vi "PPMS2 Client.vi"(8 "error in (no error)":errorcluster, 9 "Data":variant, 10 "Command":T1, 11 "instrument.PPMS2 in":refnum<class "instrument.PPMS2.lvclass">) -> (0 "error out":errorcluster, 1 "Data out":variant, 2 "Command out":string, 3 "instrument.PPMS2 out":refnum<class "instrument.PPMS2.lvclass">)   [LabVIEW 2016, in "instrument.PPMS2.lvclass"]
uses:
  instrument.PPMS2.lvclass
  C:/Program Files (x86)/National Instruments/LabVIEW 2016/user.lib/LevyLab/Levylab Instruments/SMOs/Instrument/Instrument.lvclass
  Typedefs/Commands-enum.ctl
  <userlib>/LevyLab/Levylab Instruments/SMOs/Instrument/Instrument.lvclass
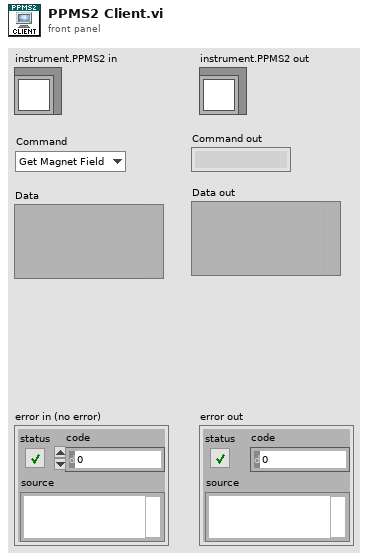
[diagram p1: front panel]
types:
  T1 = typedef "instrument.PPMS2.lvclass/Commands-enum.ctl" = enum16{"Get Magnet Field", "Get Helium Level", "Get Temperature", "Get Angle", "Set Magnet Field", "Set Temperature", "Set Angle", "getAll"}
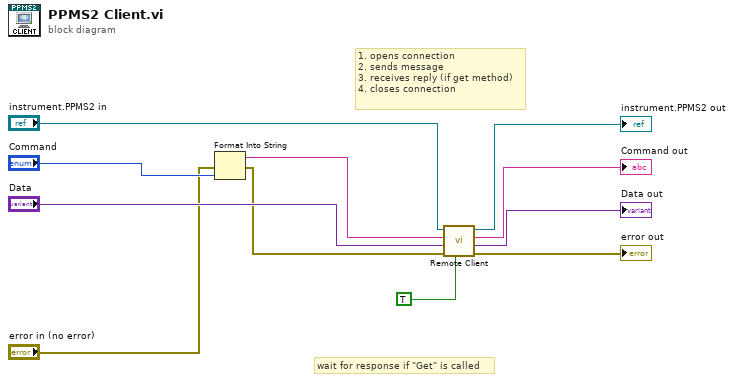
[diagram p0: block diagram]
diagram:
  # "1. opens connection\n2. sends message\n3. receives reply (if get method)\n4. closes connection"
  # "wait for response if \"Get\" is called"
  n1 = Format Into String(error in="error in (no error)", "Command") -> (resulting string=w1:string, error out=w2:errorcluster)  [unwired: 2 in]
  n2 = call <userlib>:"Remote Client.vi"("Wait for Response? [T]"=TRUE ("Wait for Response?"), "error in (no error)"=w2, "Data"="Data", "Command"=w1, "Instrument in"="instrument.PPMS2 in") -> ("error out"=→"error out":errorcluster, "Data out"=→"Data out":variant, "Command out"=→"Command out":string, "Instrument out"=→"instrument.PPMS2 out":refnum<class "instrument.PPMS2.lvclass">)  [unwired: 3 in]
